vi "Create Entity.vi"(8 "error in (no error)":errorcluster, 9 "Entity Name":string, 10 "Target Name":string, 11 "Project Name":string) -> (0 "error out":errorcluster)   [LabVIEW 2020, in "Conditum-Tools.lvlib" / "Entity Editor.lvclass"]
uses:
  Entity Editor.lvclass
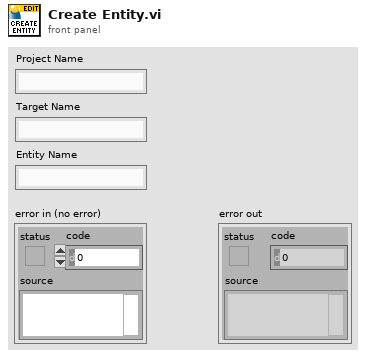
[diagram p1: front panel]
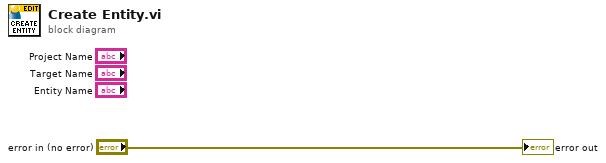
[diagram p0: block diagram]
diagram:
  "error out" <- "error in (no error)"
